vi "GetRepoContents.vi"(5 "path":string, 6 "error in":errorcluster, 8 "repo":string="LabVIEWforRasPi", 9 "owner":string="labviewforRaspi") -> (0 "error out":errorcluster, 4 "Contents":T1[](array[typedef]))   [LabVIEW 2014, in "GitHub API.lvlib"]
uses:
  GitHub API.lvlib
  TypeDefs/GitHubContents_TD.ctl
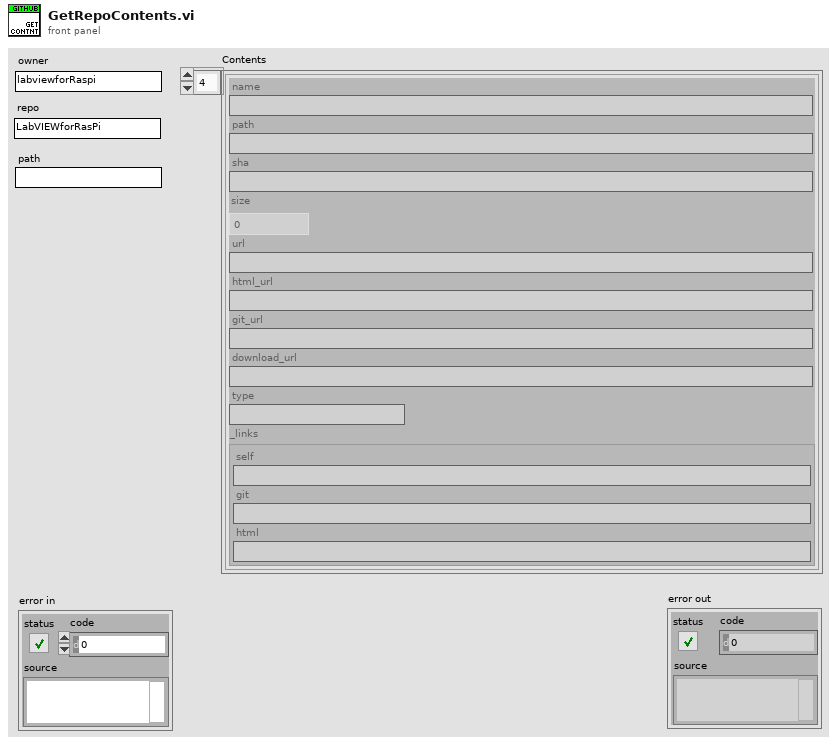
[diagram p1: front panel]
types:
  T1 = typedef "GitHub API.lvlib/GitHubContents_TD.ctl" = cluster{"name":string, "path":string, "sha":string, "size":dbl, "url":string, "html_url":string, "git_url":string, "download_url":string, "type":string, "_links":cluster{"self":string, "git":string, "html":string}}
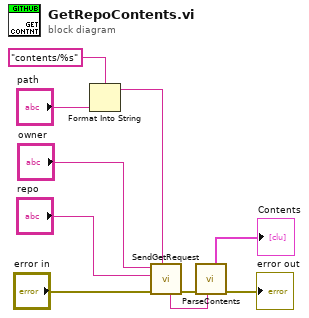
[diagram p0: block diagram]
diagram:
  n1 = Format Into String(format string="contents/%s", "path") -> (resulting string=w6:string)  [unwired: 2 in, 1 out]
  n2 = call "SendGetRequest.vi"("path"=w6, "error in"="error in", "repo"="repo", "owner"="owner") -> ("error out"=w3:errorcluster, "body"=w4:string)  [unwired: 3 in, 1 out]
  n3 = call "ParseContents.vi"("body"=w4, "error in"=w3) -> ("error out"=→"error out":errorcluster, "contents"=→"Contents":T1[])  [unwired: 6 in]
